vi "S2C_CheckSubScript.vi"(8 "Error In":errorcluster, 11 "Path":path) -> (0 "Error Out":errorcluster, 2 "Continue?":bool, 3 "Filename":string)   [LabVIEW 2015]
doc: "Adds a new blank row to the script build table if there is currently not one, and sets the Top-left cell to show the new row."
uses:
  <vilib>/Utility/config.llb/Read Key (String).vi
  <vilib>/Utility/config.llb/NI_LVConfig.lvlib
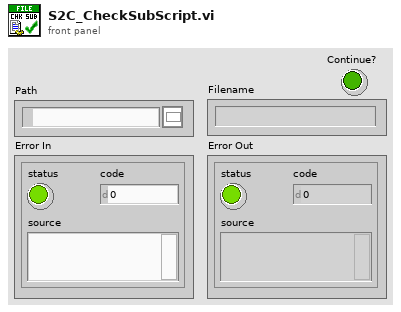
[diagram p1: front panel]
types:
  T1 = typedef "NI_LVConfig.lvlib/Config Data RefNum.ctl" = refnum<k1>
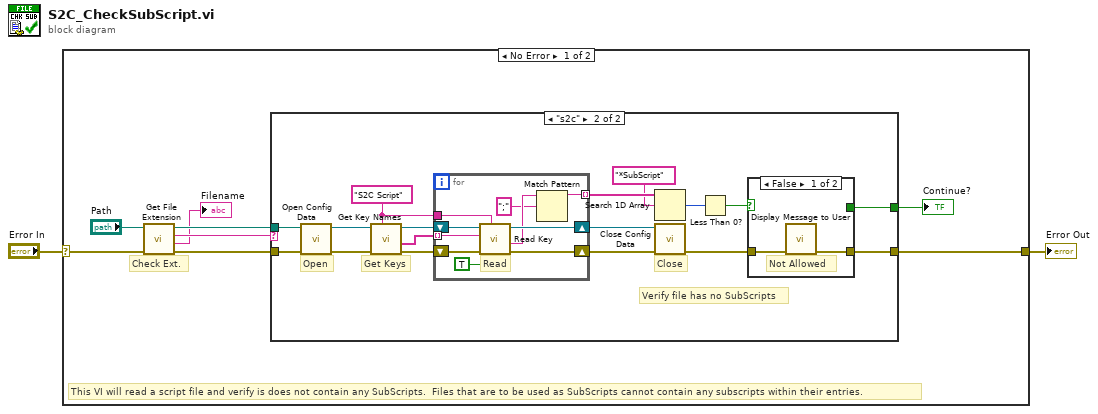
[diagram p0: block diagram]
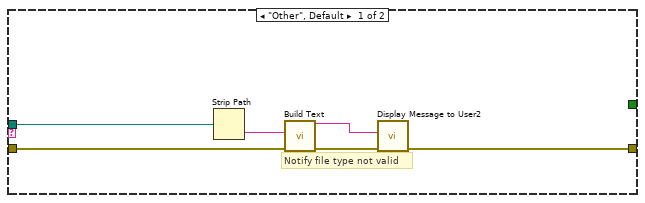
[diagram p2: hidden frame]
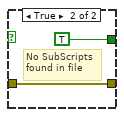
[diagram p3: hidden frame]
diagram:
  n1 = case shown="No Error" "Error In" {
    selector: "Error In" -> [w10 w48]
    tunnel: [w4 w48] -> w1
    frame No Error {
      # "This VI will read a script file and verify is does not contain any SubScripts.  Files that are to be used as SubScripts cannot contain any subscripts within their entries."
      # "Check Ext."
      n2 = call <vilib>:"Get File Extension.vi"("error in (no error)"=w10, "file"="Path") -> ("error out"=w8:errorcluster, "filename without extension"=→"Filename":string, "lowercase file extension"=w7:string, "dup file"=w9:path)  [unwired: 5 in, 1 out]
      n3 = case shown="\"s2c\"" w7 {
        tunnel: w9 -> [w11 w25]
        tunnel: w8 -> [w13 w24]
        tunnel: [w12 w18] -> w4
        tunnel: [_ w17] -> w3
        frame "Other", Default {
          # "Notify file type not valid"
          n4 = Strip Path(path=w11) -> (name=w16:string)  [unwired: 1 out]
          n5 = call "Build Text"("File"=w16, "error in (no error)"=w13) -> ("Result"=w14:string, "error out"=w15:errorcluster)  [unwired: 12 in]
          n6 = call "Display Message to User2"("error in (no error)"=w15, "Message"=w14) -> ("error out"=w12:errorcluster)  [unwired: 8 in, 1 out]
        }
        frame "s2c" {
          w28 = "S2C Script"
          # "Verify file has no SubScripts"
          # "Get Keys"
          # "Close"
          # "Open"
          n7 = call <vilib>:"Open Config Data.vi"("error in (no error)"=w24, "configuration file path"=w25) -> ("error out"=w31:errorcluster, "refnum"=w30:T1)  [unwired: 7 in, 1 out]
          n8 = call <vilib>:"Get Key Names.vi"("section"=w28, "error in (no error)"=w31, "refnum"=w30) -> ("error out"=w29:errorcluster, "key names"=w26:string[], "refnum out"=w27:T1)  [unwired: 5 in, 1 out]
          n9 = for {
            shift-right: [w41] -> w33
            shift-left: w29 -> [w47]
            tunnel: w28 -> [w46]
            shift-right: [w43] -> w32
            shift-left: w27 -> [w45]
            tunnel: w26 -> [w44] mode=indexing
            tunnel: [w38] -> w23 mode=indexing
            # "Read"
            n10 = call-poly <vilib>:"Read Key.vi"("read raw string? (F)"=TRUE, "section"=w46, "error in (no error)"=w47, "key"=w44, "refnum"=w45) -> ("error out"=w41:errorcluster, "value"=w40:string, "refnum out"=w43:T1)  [unwired: 3 in, 1 out]
            n11 = Match Pattern(string=w40, regular expression=";") -> (before substring=w38:string)  [unwired: 1 in, 3 out]
          }
          n12 = Search 1D Array(1D array=w23, element="*SubScript") -> (index of element=w21:i32)  [unwired: 1 in]
          n13 = call <vilib>:"Close Config Data.vi"("error in (no error)"=w33, "refnum"=w32) -> ("error out"=w20:errorcluster)  [unwired: 8 in, 1 out]
          n14 = Less Than 0?(x=w21) -> (x < 0?=w19:bool)
          n15 = case shown="False" w19 {
            tunnel: w20 -> [w35 w37]
            tunnel: [w34 w37] -> w18
            tunnel: [_ TRUE] -> w17
            frame False {
              # "Not Allowed"
              n16 = call "Display Message to User"("error in (no error)"=w35) -> ("error out"=w34:errorcluster)  [unwired: 9 in, 1 out]
            }
            frame True {
              # "No SubScripts\nfound in file"
            }
          }
        }
      }
      "Continue?" <- w3
    }
    frame Error {
    }
  }
  "Error Out" <- w1
